vi "Run Step.vi"(8 "error in (no error)":errorcluster, 9 "result allocation":T1, 10 "parameters":T1, 11 "Counter in":refnum<class "Counter.lvclass">) -> (0 "error out":errorcluster, 1 "results":T1, 2 "parameter allocation":T1, 3 "Counter out":refnum<class "Counter.lvclass">)   [LabVIEW 2015, in "Counter.lvclass"]
uses:
  Counter.lvclass
  <vilib>/NI/Tag Bus/table/data table.ctl
  Step/StepState.ctl
  Step/Step State Enum.ctl
  Step/Step Flow Control.ctl
  Counter.lvclass/Counter.ctl
  <vilib>/NI/Tag Bus/table/data polymorphs/write one/write Boolean.vi
  <vilib>/NI/Tag Bus/table/data polymorphs/write one/write I32.vi
  <vilib>/NI/Tag Bus/table/data table.lvlib
  Step/Step.lvclass
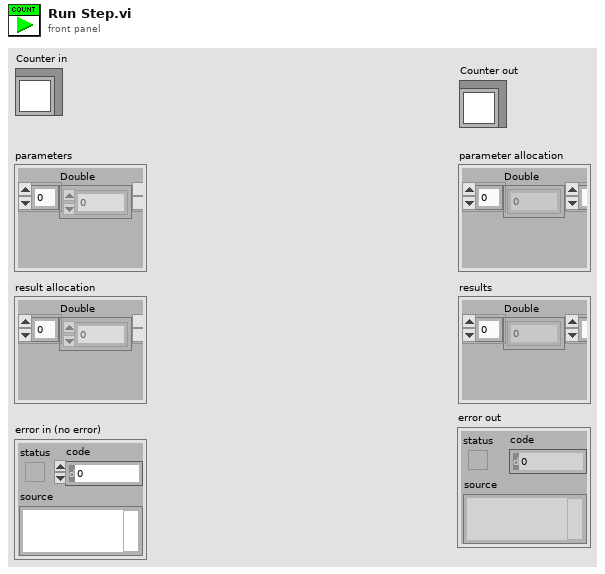
[diagram p1: front panel]
types:
  T1 = typedef "tag bus.lvlib/data table.lvlib/data table.ctl" = cluster{"Double":dbl[], "Single":sgl[], "I64":i64[], "I32":i32[], "I16":i16[], "I8":i8[], "U64":u64[], "U32":u32[], "U16":u16[], "U8":u8[], "Boolean":bool[], "String":string[], "Array of Double":cluster{"DBL Array":dbl[]}[], "Array of Single":cluster{"SGL Array":sgl[]}[], "Array of I64":cluster{"I64 Array":i64[]}[], "Array of I32":cluster{"I32 Array":i32[]}[], "Array of I16":cluster{"I16 Array":i16[]}[], "Array of I8":cluster{"I8 Array":i8[]}[], "Array of U64":cluster{"U64 Array":u64[]}[], "Array of U32":cluster{"U32 Array":u32[]}[], "Array of U16":cluster{"U16 Array":u16[]}[], "Array of U8":cluster{"U8 Array":u8[]}[], "Array of Boolean":cluster{"Boolean Array":bool[]}[], "Array of String":cluster{"String Array":string[]}[]}
  T2 = typedef "Step.lvclass/StepState.ctl" = cluster{"Step State":T3, "Flow Control":T4, "Jump Index":i32}
  T3 = typedef "Step.lvclass/Step State Enum.ctl" = enum16{"Start", "Skipped", "Completed", "Running", "Aborted"}
  T4 = typedef "Step.lvclass/Step Flow Control.ctl" = enum16{"Next Step", "Jump"}
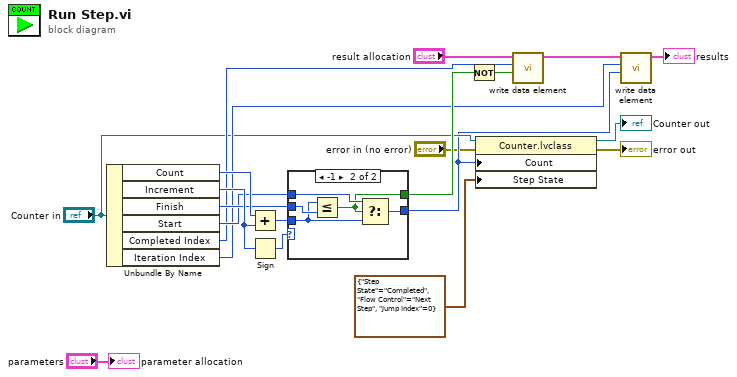
[diagram p0: block diagram]
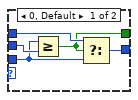
[diagram p2: hidden frame]
diagram:
  n1 = Unbundle By Name("Counter in") -> ("Count"=w20:i32, "Increment"=w19:i32, "Finish"=w17:i32, "Start"=w16:i32, "Completed Index"=w10:i32, "Iteration Index"=w9:i32)
  n2 = Add(x=w20, y=w19) -> (x+y=w15:i32)
  n3 = Sign(1:w19) -> (0:w18:i32)
  n4 = case shown="-1" w18 {
    tunnel: w15 -> [w22 w27]
    tunnel: w17 -> [w25 w30]
    tunnel: w16 -> [w24 w29]
    tunnel: [w23 w28] -> w5
    tunnel: [w21 w26] -> w11
    frame 0, Default {
      n5 = Greater Or Equal?(x=w22, y=w25) -> (x >= y?=w21:bool)
      n6 = Select(t=w24, s=w21, f=w22) -> (s? t:f=w23:i32)
    }
    frame -1 {
      n7 = Less Or Equal?(x=w27, y=w30) -> (x <= y?=w26:bool)
      n8 = Select(t=w29, s=w26, f=w27) -> (s? t:f=w28:i32)
    }
  }
  n9 = Not(x=w11) -> (.not. x?=w1:bool)
  n10 = property class="Counter.lvclass"(reference="Counter in", error in="error in (no error)", "Count"=w5, "Step State"=T2 {"Step State"=enum."Completed", "Flow Control"=enum."Next Step", "Jump Index"=0}) -> (reference out=→"Counter out":refnum<class "Counter.lvclass">, error out=→"error out":errorcluster)
  n11 = call-poly <vilib>:"write data element.vi"("value"=w1, "index"=w10, "data table in"="result allocation") -> ("data table out"=w14:T1)  [unwired: 8 in]
  n12 = call-poly <vilib>:"write data element.vi"("value"=w5, "index"=w9, "data table in"=w14) -> ("data table out"=→"results":T1)  [unwired: 8 in]
  "parameter allocation" <- "parameters"
